vi "Configure Current Limit.vi"(8 "error in (no error)":errorcluster, 10 "Current Limit":dbl, 11 "E3631A in":refnum<class "E3631A.lvclass">) -> (0 "error out":errorcluster, 3 "E3631A out":refnum<class "E3631A.lvclass">)   [LabVIEW 2020, in "E3631A.lvclass"]
uses:
  E3631A.lvclass
  C:/Sandbox/Git_Sandbox/WiSpry Test Framework source code (LV20)/WiSpry Test Framework/Instruments/Power Supply/Power Supply.lvclass
  C:/Sandbox/Git_Sandbox/WiSpry Test Framework source code (LV20)/WiSpry Test Framework/Instruments/Instrument.lvclass
  Instrument.lvclass/Instrument.ctl
  Power Supply.lvclass/Power Supply.ctl
  Instrument.lvclass
  Power Supply.lvclass
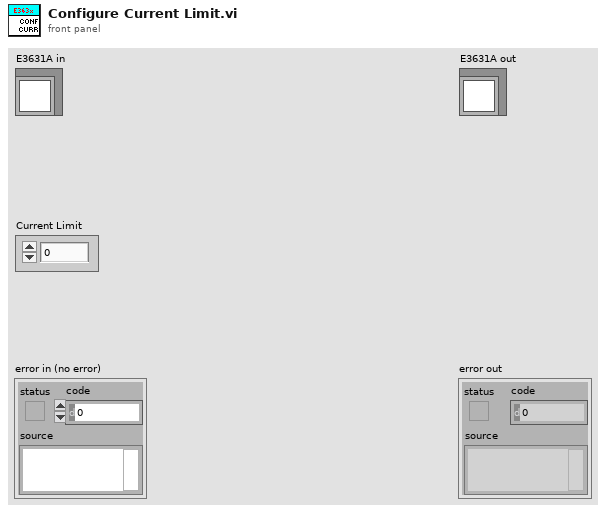
[diagram p1: front panel]
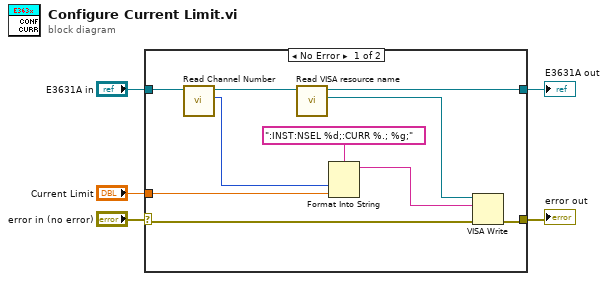
[diagram p0: block diagram]
diagram:
  n1 = case shown="No Error" "error in (no error)" {
    selector: "error in (no error)" -> [w12 w17]
    tunnel: [w13 w17] -> w4
    tunnel: "E3631A in" -> [w8 w16]
    tunnel: [w14 w16] -> w2
    tunnel: "Current Limit" -> [w9 _]
    frame No Error {
      n2 = call "Read Channel Number.vi"("Power Supply in"=w8) -> ("Channel Number"=w6:u8, "Power Supply out"=w7:refnum<class "E3631A.lvclass">)  [unwired: 9 in]
      n3 = call "Read VISA resource name.vi"("Instrument in"=w7) -> ("VISA resource name"=w15:refnum<visa-resource-name>, "Instrument out"=w14:refnum<class "E3631A.lvclass">)  [unwired: 9 in]
      n4 = Format Into String(format string=":INST:NSEL %d;:CURR %.; %g;", w6, w9) -> (resulting string=w10:string)  [unwired: 2 in, 1 out]
      n5 = VISA Write(VISA resource name=w15, write buffer=w10, error in (no error)=w12) -> (error out=w13:errorcluster)  [unwired: 2 out]
    }
    frame Error {
    }
  }
  "error out" <- w4
  "E3631A out" <- w2
